vi "WS1033 Multi Socket HD Ver1.0.vi"() -> ()   [LabVIEW 2012]
uses:
  <vilib>/Utility/file.llb/Read From Spreadsheet File (DBL).vi
  _Employee_Folders/Andy temp/All Driver/agilent/Agilent E363X Series/Agilent E363X Series.lvlib
  _Employee_Folders/Andy temp/All Driver/Keithley/keithley_2000/Keithley 2000/Keithley 2000.lvlib
panel:
  out "Simulate FPGA":bool
  out "Online":bool
  out "PS1 Out":refnum<visa-resource-name>="GPIB0::5::INSTR"
  out "Ke2000 Out":refnum<visa-resource-name>="GPIB0::9::INSTR"
  in  "Reg3&4":string[](array[string])=["0600", "0601", "0600", "0602", "0600", "0604", "0600", "0608", "0600", "0610", "0600", "0620", "0600", "0640", "0600", "0801", "0800", "0802", "0800", "0804", "0800", "0808", "0800", "0810", "0800", "06FF", "0600", "08FF", "0800"]
  in  "VPI":string[](array[string])=["0200", "02FF", "0200", "04FF", "0400", "06FF", "0600", "08FF", "0800"]
  in  "VPI Drivers":string[](array[string])=["VPI_All_Drivers OFF", "VPI_Reg1_ON", "VPI_Reg1_OFF", "VPI_Reg2_ON", "VPI_Reg2_OFF", "VPI_Reg3_ON", "VPI_Reg3_OFF", "VPI_Reg4_ON", "VPI_Reg4_OFF"]
  in  "Tab Control":enum32{"Instrument Control", "Data Output"}(tab)
  in  "CP to Hold Down":T1(ring)
  in  "VPI Test":bool=TRUE
  in  "error in (no error)":errorcluster
  out "error out":errorcluster
  in  "Lot#":string="WS1033"
  in  "Wafer#":string="T4"
  in  "File Name":string="Test Data"
  in  "TMN DC\\CAP Data Log File Path":path=path "C:/Andy Temp/16 Socket"
  in  "SN":string[](array[string])=["010", "022", "03", "04", "05", "06", "070", "08", "09", "10", "112", "12", "13", "14", "15", "160"]
  in  "Test Program":string="Multi-Sockets HD/Cycling Ver1.0"
  out "Current Date":string="5/1/2013"
  out "Current Time":string="1517"
  in  "Start Date":string
  in  "Start Time":string
  in  "Comment":string="HD at 85C"
  in  "HD/Cycles":bool=TRUE
  in  "OK Button":bool
  in  "Calibration":bool
  in  "Verify CP":bool
  in  "VSA Test":bool
  in  "Reg1_Bit Cntrl":string[](array[string])=["1", "2", "4", "8", "10", "20", "40", "80", "3", "6", "C", "D8", "33", "66", "CC", "7", "E", "1C", "38", "70", "E0", "F", "1E", "3C", "78", "F0", "1F", "3E", "7C", "F8", "3F", "7E", "FC", "7F", "FE", "FD", "FB", "F7", "EF", "DF", "BF", "7F", "FC", "F9", "F3", "E7", "CF", "9F", "3F", "F8", "F1", "E3", "C7", "8F", "1F", "F0", "E1", "C3", "87", "F", "E0", "C1", "83", "7", "C0", "81", "3", "AA", "55", "0"]
  in  "PS1 Source":refnum<visa-resource-name>="GPIB0::5::INSTR"
  in  "Ke2000":refnum<visa-resource-name>="GPIB0::9::INSTR"
  in  "CP Setting":enum16{"CP OFF", "CP ON", "CP 35V", "CP 40V"}(ring)
  out "Cap_Data":string[][](table)=[["0x02", "-0.00078", "0x02", "-0.00036"], ["0x02", "0.00029", "0x00", "-8.19200"], ["0x02", "0.00068", "0x02", "0.00013"], ["0x02", "0.00009", "0x02", "1.40700"], ["0x02", "-0.00055", "0x02", "0.00020"], ["0x02", "-0.00045", "0x02", "-0.00050"], ["0x02", "0.00012", "0x02", "-0.00015"], ["0x02", "-0.00019", "0x02", "0.00001"], ["0x02", "0.00073", "0x02", "0.00026"], ["0x02", "-0.00007", "0x02", "0.00061"], ["0x02", "0.00030", "0x02", "-0.00042"], ["0x02", "-1.44418", "0x02", "-1.41436"], ["0x02", "-0.00019", "0x02", "0.00061"], ["0x02", "-0.00016", "0x02", "0.00049"], ["0x02", "-0.00066", "0x02", "-0.00044"], ["0x02", "0.00213", "0x02", "0.00170"]]
  out "Reg3&4":string[][](table)=[["-0.00084", "0.18754", "-0.00086", "0.18760", "-0.00067", "0.38012", "-0.00140", "0.75405", "-0.00094", "0.74436", "-0.00057", "0.74920", "-0.00020", "0.71688", "-0.00073", "0.10053", "-0.00077", "0.18613", "-0.00101", "0.37569", "-0.00052", "0.73663", "-0.00098", "0.71573", "-0.00100", "3.71894", "-0.00115", "2.11771", "-0.00113"], ["-8.19200", "-8.19200", "-8.19200", "-8.19200", "-8.19200", "-8.19200", "-8.19200", "-8.19200", "-8.19200", "-8.19200", "-8.19200", "-8.19200", "-8.19200", "-8.19200", "-8.19200", "-8.19200", "-8.19200", "-8.19200", "-8.19200", "-8.19200", "-8.19200", "-8.19200", "-8.19200", "-8.19200", "-8.19200", "-8.19200", "-8.19200", "-8.19200", "-8.19200"], ["0.00018", "0.24983", "0.00031", "0.25320", "0.00005", "0.40161", "0.00013", "0.84415", "-0.00005", "0.79338", "-0.00002", "0.89156", "-0.00008", "0.78759", "-0.00012", "0.12441", "0.00009", "0.23126", "0.00023", "0.44253", "-0.00006", "0.80303", "0.00005", "0.86221", "0.00024", "4.21607", "0.00055", "2.45958", "0.00055"], ["1.48104", "1.63231", "1.48088", "1.71195", "1.48077", "1.81328", "1.48126", "2.09433", "1.48064", "2.18596", "1.48090", "2.25438", "1.48055", "2.27741", "1.48033", "1.55337", "1.48025", "1.72992", "1.48041", "1.90426", "1.48006", "2.39045", "1.48012", "2.29779", "1.48036", "5.08456", "1.48139", "3.95496", "1.48067"], ["-0.00076", "0.23402", "-0.00052", "0.23805", "0.00035", "0.43666", "-0.00035", "0.84128", "-0.00062", "0.92223", "-0.00022", "0.94897", "-0.00033", "0.81247", "-0.00029", "0.09200", "-0.00033", "0.23124", "-0.00021", "0.40000", "-0.00052", "0.89413", "-0.00028", "0.85978", "0.00024", "4.43176", "0.00034", "2.47569", "0.00022"], ["0.00009", "0.18310", "-0.00025", "0.20594", "-0.00012", "0.36049", "-0.00083", "0.75674", "-0.00085", "0.80900", "0.00001", "0.77914", "-0.00048", "0.72434", "-0.00073", "0.10624", "-0.00040", "0.21135", "-0.00031", "0.39919", "-0.00078", "0.80036", "0.00025", "0.78208", "-0.00029", "3.81718", "-0.00030", "2.30191", "-0.00016"], ["0.00018", "0.23801", "0.00002", "0.20572", "0.00043", "0.45364", "0.00013", "0.85310", "0.00030", "0.88533", "0.00002", "0.86306", "0.00027", "0.90155", "0.00011", "0.11996", "0.00020", "0.20562", "0.00029", "0.38279", "-0.00007", "0.82877", "0.00010", "0.84844", "0.00000", "4.39414", "0.00041", "2.38263", "0.00046"], ["-0.00025", "-0.00033", "-0.00033", "-0.00005", "-0.00034", "-0.00020", "-0.00026", "-0.00016", "-0.00029", "-0.00028", "-0.00036", "-0.00026", "-0.00022", "0.00003", "-0.00031", "-0.00006", "-0.00004", "-0.00028", "-0.00012", "0.00002", "-0.00038", "-0.00007", "-0.00022", "-0.00013", "-0.00006", "0.00002", "0.00004", "-0.00006", "-0.00028"], ["-0.00024", "0.22994", "-0.00010", "0.20515", "0.00022", "0.35799", "0.00006", "0.85993", "0.00025", "0.49771", "-0.00013", "0.87203", "0.00013", "0.85128", "-0.00010", "0.10478", "-0.00009", "0.17132", "-0.00025", "0.27951", "0.00002", "0.88446", "-0.00001", "0.80268", "0.00025", "3.87229", "0.00045", "2.24245", "0.00032"], ["-0.00000", "0.21432", "0.00055", "0.22416", "0.00066", "0.46476", "0.00079", "0.82063", "0.00088", "0.91417", "0.00085", "0.71087", "0.00137", "0.88451", "0.00047", "0.12494", "0.00100", "0.21354", "0.00111", "0.39845", "0.00135", "0.87188", "0.00073", "0.83177", "0.00040", "4.22709", "0.00114", "2.43520", "0.00173"], ["0.00004", "0.21202", "0.00087", "0.18791", "-0.00050", "0.37207", "0.00000", "0.77774", "0.00003", "0.76047", "-0.00026", "0.73879", "0.00033", "0.74256", "0.00113", "0.09446", "-0.00033", "0.20280", "0.00057", "0.40386", "-0.00006", "0.74892", "0.00009", "0.75346", "0.00005", "3.78760", "-0.00022", "2.20027", "0.00007"], ["-1.38608", "-1.41365", "-1.38569", "-1.40262", "-1.41280", "-1.38552", "-1.38403", "-1.40605", "-1.41116", "-1.40218", "-1.38437", "-1.39281", "-1.41380", "-1.38576", "-1.41076", "-1.41382", "-1.38948", "-1.38451", "-1.40341", "-1.41316", "-1.38565", "-1.38617", "-1.41285", "-1.38543", "-1.39807", "-1.41301", "-1.38564", "-1.38315", "-1.41346"], ["-0.00011", "-0.00018", "-0.00016", "-0.00032", "0.00006", "0.00022", "-0.00012", "0.00029", "-0.00018", "-0.00014", "-0.00028", "-0.00016", "-0.00028", "-0.00043", "-0.00018", "-0.00058", "-0.00030", "-0.00043", "-0.00003", "-0.00086", "0.00001", "-0.00024", "-0.00032", "-0.00022", "-0.00052", "-0.00009", "-0.00015", "-0.00018", "-0.00010"], ["-0.28766", "-0.06844", "-0.28721", "-0.07378", "-0.28779", "0.09271", "-0.28773", "0.52467", "-0.28712", "0.47110", "-0.28710", "0.42933", "-0.31981", "0.48753", "-0.30479", "-0.19809", "-0.30441", "-0.09968", "-0.30354", "0.09009", "-0.30382", "0.49702", "-0.30349", "0.09602", "-0.30717", "3.60367", "-0.25810", "1.64223", "-0.25957"], ["-0.00059", "0.19570", "-0.00082", "0.20174", "0.00001", "0.39111", "-0.00072", "0.75114", "-0.00106", "0.76788", "-0.00014", "0.77680", "-0.00006", "0.76978", "-0.00018", "0.10645", "-0.00070", "0.20429", "-0.00002", "0.37780", "-0.00030", "0.81574", "-0.00013", "0.47817", "-0.00074", "3.85303", "-0.00048", "1.98246", "-0.00087"], ["0.00088", "0.20894", "-0.00005", "0.22869", "-0.00426", "0.43002", "0.00310", "0.90978", "-0.00419", "0.79785", "-0.00166", "0.91643", "0.00103", "0.78807", "0.00092", "0.11746", "-0.00434", "0.23011", "0.00081", "0.44810", "0.00235", "0.85701", "-0.00171", "0.69913", "-0.00388", "4.28342", "-0.00044", "2.35229", "0.00221"]]
  out "Reg1&2":string[][](table)=[["-0.00108", "0.08958", "-0.00053", "0.18959", "-0.00078", "0.37850", "-0.00171", "0.76297", "-0.00120", "0.76690", "-0.00101", "0.77762", "-0.00044", "0.77961", "-0.00083", "0.18983", "-0.00150", "0.19728", "-0.00157", "0.36782", "-0.00119", "0.75459", "-0.00103", "0.71258", "-0.00099", "3.74809", "-0.00130", "2.22378", "-0.00086"], ["-0.00041", "0.10906", "-0.00055", "0.19752", "-0.00042", "0.45314", "-0.00099", "0.87667", "-0.00092", "0.86594", "-0.00012", "0.87358", "-0.00063", "0.85050", "-0.00091", "0.19742", "-0.00169", "0.22081", "-0.00095", "0.43763", "-0.00006", "0.81361", "0.00021", "0.79624", "0.00004", "4.22385", "-0.00056", "2.46734", "0.00029"], ["-0.00071", "0.12205", "-0.00101", "0.23127", "-0.00120", "0.45826", "-0.00166", "0.76407", "-0.00138", "0.93942", "-0.00113", "0.85225", "-0.00202", "0.71053", "-0.00199", "0.18763", "-0.00186", "0.20697", "-0.00161", "0.45450", "-0.00214", "0.91461", "-0.00233", "0.89898", "-0.00220", "4.07969", "-0.00177", "2.66987", "-0.00206"], ["0.00302", "0.12120", "0.00300", "0.23274", "0.00271", "0.43565", "0.00310", "0.81019", "0.00284", "0.80161", "0.00285", "0.85918", "0.00327", "0.75798", "0.00290", "0.17085", "0.00258", "0.26002", "0.00243", "0.36001", "0.00210", "0.84827", "0.00265", "0.83634", "0.00302", "3.99829", "0.00392", "2.46160", "0.00326"], ["-0.00053", "0.10355", "0.00018", "0.23057", "-0.00018", "0.41330", "-0.00084", "0.85901", "-0.00029", "0.90795", "-0.00049", "0.86511", "-0.00023", "0.66685", "-0.00013", "0.20790", "-0.00045", "0.23230", "-0.00036", "0.36861", "-0.00021", "0.91175", "-0.00039", "0.89470", "-0.00022", "4.04444", "0.00030", "2.61219", "0.00067"], ["-0.00065", "0.10915", "-0.00041", "0.15397", "-0.00086", "0.40657", "-0.00049", "0.80189", "-0.00024", "0.79573", "-0.00090", "0.74982", "0.00009", "0.74729", "-0.00032", "0.20103", "-0.00066", "0.15526", "-0.00050", "0.35926", "-0.00085", "0.76617", "-0.00037", "0.73687", "-0.00084", "3.76376", "0.00006", "2.21866", "-0.00009"], ["0.00030", "0.12056", "0.00004", "0.20153", "0.00009", "0.42879", "0.00031", "0.89839", "0.00030", "0.70209", "0.00002", "0.88332", "-0.00002", "0.93653", "-0.00001", "0.23214", "0.00040", "0.24748", "0.00040", "0.38589", "-0.00015", "0.75535", "0.00037", "0.89693", "0.00052", "4.16809", "0.00050", "2.51317", "0.00018"], ["0.00012", "-0.00046", "-0.00024", "-0.00022", "-0.00021", "0.00039", "0.00039", "0.00026", "0.00009", "0.00010", "-0.00005", "0.00003", "-0.00016", "0.00013", "-0.00015", "0.00033", "0.00036", "0.00017", "0.00032", "0.00028", "0.00018", "0.00043", "-0.00002", "0.00009", "0.00019", "0.00002", "0.00005", "0.00006", "-0.00005"], ["0.00070", "0.11336", "0.00036", "0.21945", "-0.00001", "0.38795", "0.00026", "0.82826", "0.00041", "0.80312", "-0.00028", "0.40543", "0.00037", "0.75070", "0.00052", "0.18489", "-0.00025", "0.21492", "0.00034", "0.43130", "0.00022", "0.86169", "0.00032", "0.82752", "0.00056", "3.50231", "0.00059", "2.51767", "0.00054"], ["-0.00061", "0.09307", "-0.00031", "0.17837", "-0.00027", "0.43916", "-0.00046", "0.88525", "-0.00032", "0.82577", "-0.00056", "0.86653", "-0.00034", "0.90515", "-0.00020", "0.20958", "-0.00047", "0.20748", "-0.00045", "0.46265", "-0.00032", "0.90088", "-0.00056", "0.79231", "-0.00016", "4.19054", "0.00021", "2.57487", "0.00006"], ["0.00103", "0.10551", "0.00060", "0.20551", "0.00094", "0.32942", "0.00117", "0.71118", "0.00014", "0.76176", "0.00086", "0.80010", "0.00036", "0.75930", "0.00082", "0.18517", "0.00065", "0.21107", "0.00123", "0.37059", "0.00126", "0.74420", "-0.00022", "0.71578", "0.00077", "3.66523", "0.00031", "2.22177", "0.00081"], ["-1.42429", "-1.44113", "-1.41095", "-1.44427", "-1.44315", "-1.41113", "-1.41886", "-1.44365", "-1.44414", "-1.42234", "-1.41414", "-1.43293", "-1.44072", "-1.41408", "-1.44534", "-1.44074", "-1.41168", "-1.41344", "-1.44284", "-1.44325", "-1.41192", "-1.42341", "-1.44250", "-1.41447", "-1.43829", "-1.44336", "-1.41174", "-1.41548", "-1.44290"], ["-0.00040", "-0.00058", "-0.00069", "-0.00034", "-0.00091", "-0.00007", "-0.00026", "0.00017", "-0.00029", "-0.00053", "-0.00067", "-0.00019", "-0.00032", "-0.00082", "-0.00022", "-0.00101", "-0.00044", "-0.00060", "-0.00033", "-0.00070", "-0.00014", "-0.00033", "-0.00039", "-0.00033", "-0.00050", "-0.00045", "-0.00058", "-0.00057", "-0.00050"], ["0.26147", "0.37198", "0.26509", "0.37993", "0.26735", "0.61084", "0.27247", "1.16162", "0.35145", "0.37885", "0.19776", "0.31024", "0.20096", "0.87044", "0.12135", "0.33067", "0.12190", "0.31888", "0.12124", "0.49791", "0.12085", "0.83089", "0.11981", "0.90413", "0.12004", "2.33768", "0.36618", "2.64833", "0.37380"], ["-0.00125", "0.08024", "-0.00154", "0.18501", "-0.00112", "0.35777", "-0.00077", "0.79151", "-0.00136", "0.70398", "-0.00169", "0.76332", "-0.00093", "0.74859", "-0.00069", "0.17705", "-0.00076", "0.16984", "-0.00130", "0.38821", "-0.00132", "0.79636", "-0.00084", "0.74254", "-0.00106", "3.63462", "-0.00039", "2.27469", "-0.00088"], ["-0.00006", "0.10215", "0.00384", "0.20083", "-0.00340", "0.41008", "0.00403", "0.77711", "-0.00457", "0.89558", "0.00300", "0.84232", "0.00019", "0.89071", "0.00511", "0.24260", "-0.00298", "0.23605", "0.00029", "0.35134", "0.00335", "0.77986", "0.00245", "0.86336", "-0.00354", "4.12034", "-0.00111", "2.46775", "0.00576"]]
  out "STATUS":string="Idle...."
  in  "Set HD/Cycle \nto Complete":i16=2
  out "No of HD/Cycle\nCompleted":i16=2
  out "EFuse Readback Status":bool[](array[boolean])
  in  "stop During HD/Cycles":bool
  in  "stop":bool
  in  "Reg1&2":string[](array[string])=["0200", "0201", "0200", "0202", "0200", "0204", "0200", "0208", "0200", "0210", "0200", "0220", "0200", "0240", "0200", "0401", "0400", "0402", "0400", "0404", "0400", "0408", "0400", "0410", "0400", "02FF", "0200", "04FF", "0400"]
  in  "Drivers":string[](array[string])=["C1_1 & C2_1Min", "C1_D0 & C2_D12", "C1_D0 & C2_D12 OFF", "C1_D1 & C2_D13", "C1_D1 & C2_D13 OFF", "C1_D2 & C2_D14", "C1_D2 & C2_D14 OFF", "C1_D3 & C2_D15", "C1_D3 & C2_D15 OFF", "C1_D4 & C2_D16", "C1_D4 & C2_D16 OFF", "C1_D5 & C2_D17", "C1_D5 & C2_D17 OFF", "C1_D6 & C2_D18", "C1_D6 & C2_D18 OFF", "C1_D7 & C2_D19", "C1_D7 & C2_D19 OFF", "C1_D8 & C2_D20", "C1_D8 & C2_D20 OFF", "C1_D9 & C2_D21", "C1_D9 & C2_D21 OFF", "C1_D10 & C2_D22", "C1_D10 & C2_D22 OFF", "C1_D11 & C2_D23", "C1_D11 & C2_D23 OFF", "Reg1 & Reg3 ON", "Reg1 & Reg3 OFF", "Reg2 & Reg4 ON", "Reg2 & Reg4 OFF"]
  # "*********** Do Not Remove*******\nCompany:  WiSpry Inc\n20 Fairbanks Ste 198 Irvine CA 92618\n\nAuthor:  Andy V Tran\nCreated:  03/06/2013\nLabVIEW2009 Pro\nTest Program:  \nWS1033 Multi-Socket HD/Cycle ver1.0\n*******************************"
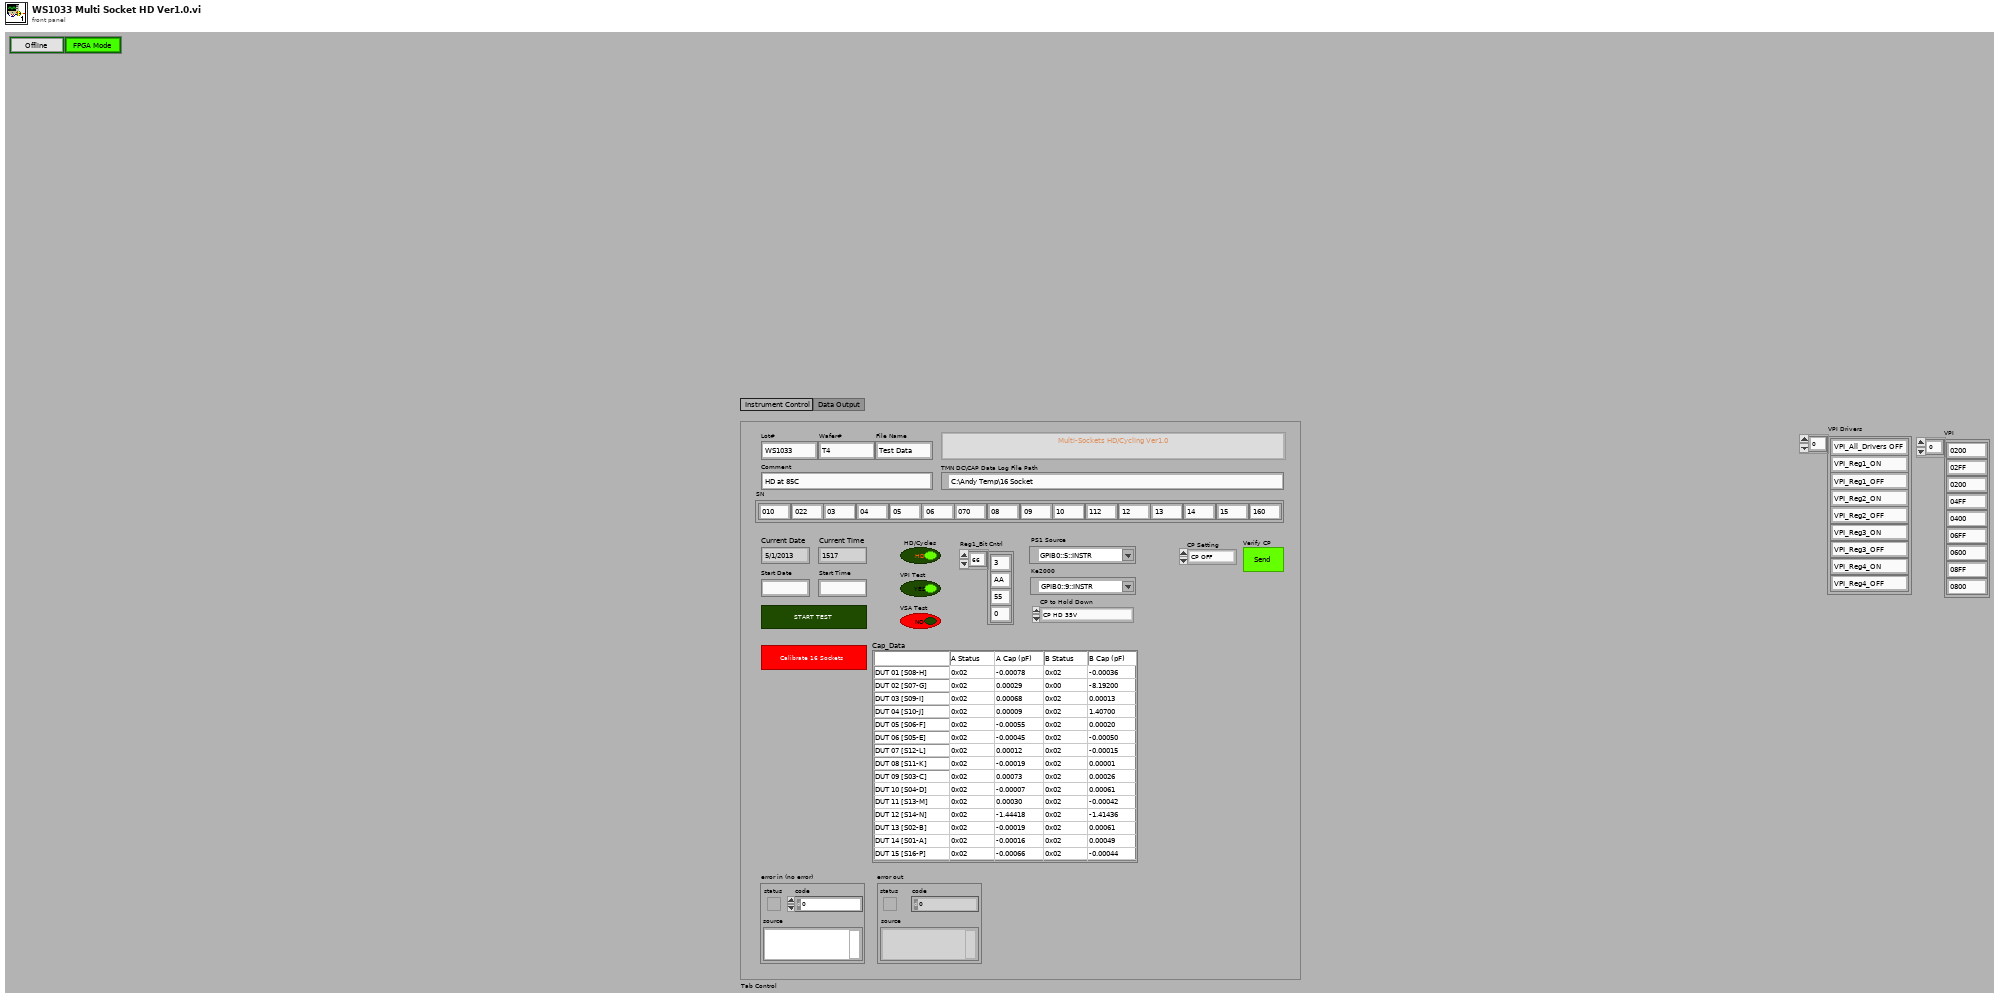
[diagram p1: front panel]
types:
  T1 = enum16{"CP HD 35V", "CP HD 40V", "CP HD 26V", "CP HD 30V"}
  T2 = typedef "WSVCAP SHL Core System Cluster.ctl" = cluster{"Settings":T3, "FPGA Resource":tag, "Online":bool}
  T3 = typedef "WSVCAP SHL I2C Settings Cluster.ctl" = cluster{"FPGA Resource Name":string, "I2C Slave Address":u8, "I2C Clock Rate (Hz)":dbl, "SPI Clock Rate (Hz)":dbl, "Simulate FPGA":bool}
  T4 = enum16{"Idle...", "Voltage 1", "Voltage 2", "Voltage 3"}[]
  T5 = cluster{"Test Program ":string, "Comment":string}
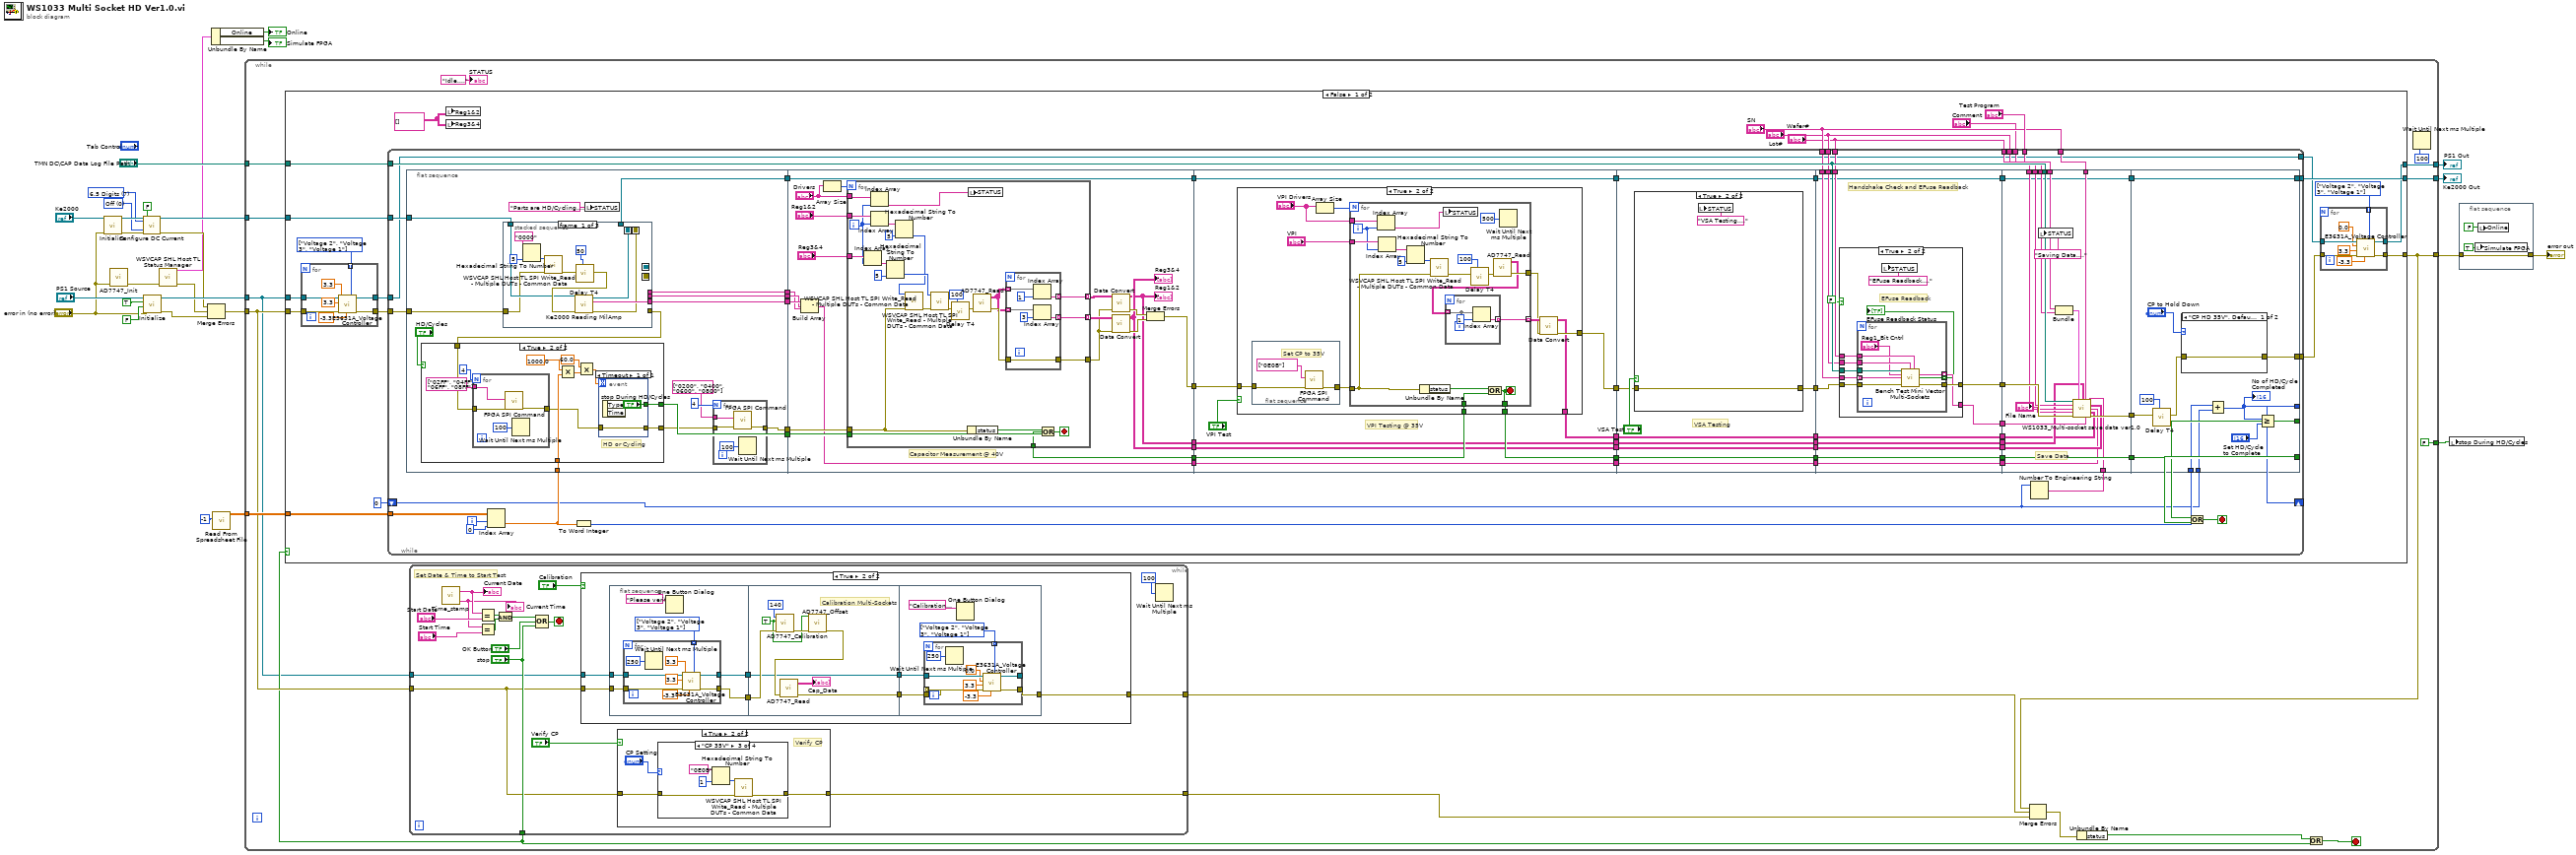
[diagram p0: block diagram]
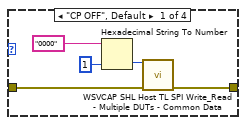
[diagram p3: hidden frame]
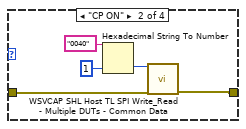
[diagram p4: hidden frame]
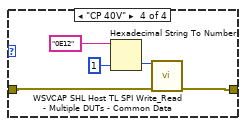
[diagram p5: hidden frame]
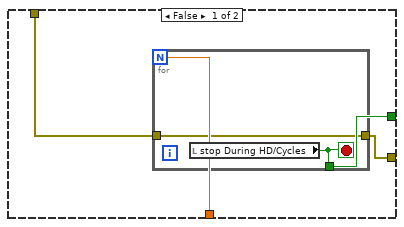
[diagram p7: hidden frame]
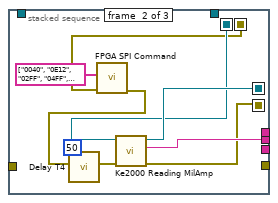
[diagram p8: hidden frame]
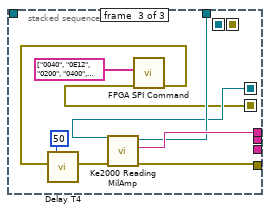
[diagram p9: hidden frame]
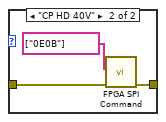
[diagram p13: hidden frame]
diagram:
  w17 = u16 0 items=["Off", "Moving Filter", "Repeating Filter"] ("Digital Filter (0: Off)")
  w18 = u16 7 items=["3.5 Digits"=4, "4.5 Digits"=5, "5.5 Digits"=6, "6.5 Digits"=7] ("Resolution (7: 6.5 digits)")
  n1 = call "Initialize.vi"("VISA resource name"="Ke2000", "error in (no error)"="error in (no error)") -> ("VISA resource name out"=w20:refnum<visa-resource-name>, "error out"=w19:errorcluster)  [unwired: 16 in]
  n2 = call "AD7747_Init.vi"("error in"="error in (no error)") -> ("error out"=w4:errorcluster)  [unwired: 10 in]
  n3 = call "Configure DC Current.vi"("VISA resource name"=w20, "Resolution (7: 6.5 digits)"=w18, "error in (no error)"=w19, "Auto Range? (T: Auto)"=FALSE, "Digital Filter (0: Off)"=w17) -> ("VISA resource name out"=w11:refnum<visa-resource-name>, "error out"=w14:errorcluster)  [unwired: 13 in]
  n4 = call "Initialize.vi"("error in (no error)"="error in (no error)", "Reset? (T: Yes)"=FALSE, "ID Query? (T: Yes)"=TRUE, "VISA resource name"="PS1 Source") -> ("error out"=w13:errorcluster, "VISA resource name out"=w23:refnum<visa-resource-name>)  [unwired: 6 in]
  n5 = call "WSVCAP SHL Host TL Status Manager.vi"("error in"=w4) -> ("System Out"=w7:T2, "error out"=w3:errorcluster)  [unwired: 13 in]
  n6 = Merge Errors(w14, w3, w13) -> (w12:errorcluster)
  n7 = Unbundle By Name(w7) -> ("Online"=→"Online":bool, "Settings.Simulate FPGA"=→"Simulate FPGA":bool)
  n8 = call-poly <vilib>:"Read From Spreadsheet File.vi"("number of rows (all:-1)"=-1) -> ("all rows"=w27:dbl[][])  [unwired: 6 in, 4 out]
  n9 = while {
    tunnel: w12 -> [w39]
    tunnel: [w37] -> w1
    tunnel: w27 -> [w42]
    tunnel: "TMN DC\\CAP Data Log File Path" -> [w41]
    tunnel: w23 -> [w33]
    tunnel: w11 -> [w32]
    tunnel: [w31] -> w10
    tunnel: [w30] -> w9
    tunnel: [FALSE ("stop During HD/Cycles")] -> w8
    stop <- w43 stop-if-true
    n10 = while {
      tunnel: ["stop"] -> w38
      tunnel: w39 -> [w49]
      tunnel: [w48] -> w36
      tunnel: [w47] -> w35
      tunnel: w33 -> [w46]
      stop <- w55 stop-if-true
      # "Set Date & Time to Start Test"
      n11 = call "Time_stamp.vi"() -> ("date/time string"=w60:string, "date string"=w62:string)  [unwired: 2 in]
      "Current Date" <- w62
      "Current Time" <- w60
      n12 = Equal?(x=w62, y="Start Date") -> (x = y?=w58:bool)
      n13 = Equal?(x=w60, y="Start Time") -> (x = y?=w57:bool)
      n14 = And(x=w58, y=w57) -> (x .and. y?=w54:bool)
      n15 = Compound Arithmetic op=OR(w54, "OK Button", "stop") -> (w55:bool)
      n16 = case shown="True" "Calibration" {
        tunnel: w49 -> [w87 w94]
        tunnel: [w87 w91] -> w48
        tunnel: w46 -> [_ w90]
        frame False {
        }
        frame True {
          n17 = flat-sequence {
            tunnel: w94 -> [w98]
            tunnel: [w97] -> w93
            tunnel: w90 -> [w96]
            tunnel: [w95] -> w89
            tunnel: w93 -> [w115]
            tunnel: [w112] -> w92
            tunnel: w89 -> [w110]
            tunnel: [w110] -> w88
            tunnel: w92 -> [w120]
            tunnel: [w121] -> w91
            tunnel: w88 -> [w119]
            frame #0 {
              w99 = T4 [enum."Voltage 2", enum."Voltage 3", enum."Voltage 1"] items=["Idle...", "Voltage 1", "Voltage 2", "Voltage 3"]
              n18 = for {
                tunnel: w98 -> [w109]
                tunnel: w96 -> [w108]
                tunnel: w99 -> [w104] mode=indexing
                tunnel: [w103] -> w97
                tunnel: [w102] -> w95
                n19 = Wait Until Next ms Multiple(millisecond multiple=u32 250) -> ()  [unwired: 1 out]
                n20 = call "E3631A_Voltage Controller.vi"("Channel Controller"=w104, "Voltage 3"=-3.3, "error in (no error)"=w109, "Voltage 2"=3.3, "Voltage 1"=3.3, "VISA resource name"=w108) -> ("error out"=w103:errorcluster, "VISA resource name out"=w102:refnum<visa-resource-name>)  [unwired: 4 in]
              }
              n21 = One Button Dialog(message="Please verify all sockets should be empty...") -> ()  [unwired: 1 in, 1 out]
            }
            frame #1 {
              w114 = TRUE ("Read After CapDac?")
              # "Calibration Multi-Sockets"
              n22 = call "AD7747_Calibration.vi"("error in"=w115, "Read After CapDac?"=w114, "Cap_Dac Value"=u8 140) -> ("errorout"=w116:errorcluster)  [unwired: 7 in, 1 out]
              n23 = call "AD7747_Offset.vi"("error in"=w116, "Read?"=w114) -> ("error Out"=w113:errorcluster)  [unwired: 8 in, 1 out]
              n24 = call "AD7747_Read.vi"("error in"=w113) -> ("error Out"=w112:errorcluster, "AD7747 Values"=→"Cap_Data":string[][])  [unwired: 3 in]
            }
            frame #2 {
              w118 = T4 [enum."Voltage 2", enum."Voltage 3", enum."Voltage 1"] items=["Idle...", "Voltage 1", "Voltage 2", "Voltage 3"]
              n25 = for {
                tunnel: [w124] -> _ mode=indexing
                tunnel: w119 -> [w131]
                tunnel: w118 -> [w123] mode=indexing
                tunnel: [w127] -> w121
                tunnel: [w126] -> _
                tunnel: w120 -> [w124]
                n26 = Wait Until Next ms Multiple(millisecond multiple=u32 250) -> ()  [unwired: 1 out]
                n27 = call "E3631A_Voltage Controller.vi"("Channel Controller"=w123, "Voltage 3"=-3.3, "error in (no error)"=w124, "Voltage 2"=3.3, "Voltage 1"=0.0, "VISA resource name"=w131) -> ("error out"=w127:errorcluster, "VISA resource name out"=w126:refnum<visa-resource-name>)  [unwired: 4 in]
              }
              n28 = One Button Dialog(message="Calibration Completed....") -> ()  [unwired: 1 in, 1 out]
            }
          }
        }
      }
      n29 = case shown="True" "Verify CP" {
        tunnel: w49 -> [w63 w66]
        tunnel: [w63 w65] -> w47
        frame False {
        }
        frame True {
          # "Verify CP"
          n30 = case shown="\"CP 35V\"" "CP Setting" {
            tunnel: w66 -> [w69 w74 w78 w83]
            tunnel: [w68 w73 w79 w84] -> w65
            frame "CP OFF", Default {
              n31 = Hexadecimal String To Number(string="0000" ("SPI Command"), default (0uL)=u16 1 ("default (0 U32)")) -> (number=w71:u16)  [unwired: 1 in, 1 out]
              n32 = call "WSVCAP SHL Host TL SPI Write_Read - Multiple DUTs - Common Data.vi"("Data Out [U64]"=w71, "error in"=w69) -> ("error out"=w68:errorcluster)  [unwired: 12 in, 1 out]
            }
            frame "CP ON" {
              n33 = Hexadecimal String To Number(string="0040" ("SPI Command"), default (0uL)=u16 1 ("default (0 U32)")) -> (number=w76:u16)  [unwired: 1 in, 1 out]
              n34 = call "WSVCAP SHL Host TL SPI Write_Read - Multiple DUTs - Common Data.vi"("Data Out [U64]"=w76, "error in"=w74) -> ("error out"=w73:errorcluster)  [unwired: 12 in, 1 out]
            }
            frame "CP 35V" {
              n35 = Hexadecimal String To Number(string="0E0B" ("SPI Command"), default (0uL)=u16 1 ("default (0 U32)")) -> (number=w81:u16)  [unwired: 1 in, 1 out]
              n36 = call "WSVCAP SHL Host TL SPI Write_Read - Multiple DUTs - Common Data.vi"("Data Out [U64]"=w81, "error in"=w78) -> ("error out"=w79:errorcluster)  [unwired: 12 in, 1 out]
            }
            frame "CP 40V" {
              n37 = Hexadecimal String To Number(string="0E12" ("SPI Command"), default (0uL)=u16 1 ("default (0 U32)")) -> (number=w86:u16)  [unwired: 1 in, 1 out]
              n38 = call "WSVCAP SHL Host TL SPI Write_Read - Multiple DUTs - Common Data.vi"("Data Out [U64]"=w86, "error in"=w83) -> ("error out"=w84:errorcluster)  [unwired: 12 in, 1 out]
            }
          }
        }
      }
      n39 = Wait Until Next ms Multiple(millisecond multiple=u32 100) -> ()  [unwired: 1 out]
    }
    n40 = case shown="False" w38 {
      tunnel: w39 -> [w144 w481]
      tunnel: [w133 w481] -> w37
      tunnel: w42 -> [w151 _]
      tunnel: w41 -> [w150 _]
      tunnel: w33 -> [w143 w479]
      tunnel: w32 -> [w140 w480]
      tunnel: [w139 w480] -> w31
      tunnel: [w135 w479] -> w30
      frame False {
        w132 = string[][] []
        w137 = T4 [enum."Voltage 2", enum."Voltage 3", enum."Voltage 1"] items=["Idle...", "Voltage 1", "Voltage 2", "Voltage 3"]
        w142 = T4 [enum."Voltage 2", enum."Voltage 3", enum."Voltage 1"] items=["Idle...", "Voltage 1", "Voltage 2", "Voltage 3"]
        n41 = for {
          tunnel: w144 -> [w168]
          tunnel: w143 -> [w167]
          tunnel: w142 -> [w163] mode=indexing
          tunnel: [w162] -> w141
          tunnel: [w161] -> w138
          n42 = call "E3631A_Voltage Controller.vi"("Channel Controller"=w163, "Voltage 3"=-3.3, "error in (no error)"=w168, "Voltage 2"=3.3, "Voltage 1"=3.3, "VISA resource name"=w167) -> ("error out"=w162:errorcluster, "VISA resource name out"=w161:refnum<visa-resource-name>)  [unwired: 4 in]
        }
        n43 = while {
          tunnel: w141 -> [w207]
          tunnel: [w223] -> w134
          tunnel: w151 -> [w230]
          shift-right: [w173] -> _
          shift-left: i16 0 -> [w169]
          tunnel: w150 -> [w217]
          tunnel: "Lot#" -> [w216]
          tunnel: "Wafer#" -> [w215]
          tunnel: "SN" -> [w214]
          tunnel: "Test Program" -> [w213]
          tunnel: "SN" -> [w212]
          tunnel: "Comment" -> [w211]
          tunnel: "Lot#" -> [w210]
          tunnel: "Wafer#" -> [w209]
          tunnel: w140 -> [w204]
          tunnel: [w198] -> w139
          tunnel: w138 -> [w197]
          tunnel: [w197] -> w136
          i -> [w228]
          stop <- w229 stop-if-true
          n44 = flat-sequence {
            tunnel: w170 -> [w245]
            tunnel: [w244] -> w226
            tunnel: w207 -> [w243]
            tunnel: [w234] -> w224
            tunnel: w204 -> [w239]
            tunnel: [w238] -> w203
            tunnel: [w237] -> w196
            tunnel: [w236] -> w195
            tunnel: [w235] -> w194
            tunnel: w226 -> [w320]
            tunnel: [w318] -> w192
            tunnel: w224 -> [w319]
            tunnel: [w305] -> w191
            tunnel: w203 -> [w314]
            tunnel: [w314] -> w190
            tunnel: w196 -> [w313]
            tunnel: w195 -> [w312]
            tunnel: w194 -> [w311]
            tunnel: [w304] -> w189
            tunnel: [w303] -> w188
            tunnel: [w302] -> w181
            tunnel: [w360] -> w222
            tunnel: [w359] -> w202
            tunnel: [w358] -> w193
            tunnel: w190 -> [w359]
            tunnel: w191 -> [w357]
            tunnel: w192 -> [w361]
            tunnel: w189 -> [w355]
            tunnel: w188 -> [w356]
            tunnel: [w356] -> w187
            tunnel: [w355] -> w186
            tunnel: w181 -> [w354]
            tunnel: [w354] -> w180
            tunnel: [w353] -> w176
            tunnel: w222 -> [w407]
            tunnel: [w407] -> w221
            tunnel: [w405] -> w219
            tunnel: w202 -> [w404]
            tunnel: [w404] -> w201
            tunnel: w193 -> [w403]
            tunnel: w187 -> [w402]
            tunnel: w186 -> [w401]
            tunnel: [w402] -> w185
            tunnel: [w401] -> w184
            tunnel: w180 -> [w400]
            tunnel: [w400] -> w179
            tunnel: w176 -> [w399]
            tunnel: [w399] -> w175
            tunnel: w221 -> [w424]
            tunnel: [w424] -> w220
            tunnel: w219 -> [w422]
            tunnel: [w421] -> w218
            tunnel: w217 -> [w423]
            tunnel: w216 -> [w420]
            tunnel: w215 -> [w419]
            tunnel: w214 -> [w418]
            tunnel: [w417] -> w208
            tunnel: w201 -> [w416]
            tunnel: [w416] -> w200
            tunnel: w185 -> [w414]
            tunnel: w184 -> [w413]
            tunnel: [w414] -> w183
            tunnel: [w413] -> w182
            tunnel: w179 -> [w412]
            tunnel: [w412] -> w178
            tunnel: w175 -> [w411]
            tunnel: [w411] -> w174
            tunnel: w220 -> [w462]
            tunnel: w218 -> [w461]
            tunnel: w217 -> [w459]
            tunnel: w213 -> [w453]
            tunnel: w212 -> [w457]
            tunnel: w211 -> [w452]
            tunnel: w210 -> [w456]
            tunnel: w209 -> [w451]
            tunnel: w208 -> [w454]
            tunnel: [w462] -> w206
            tunnel: [w460] -> w205
            tunnel: w200 -> [w449]
            tunnel: [w449] -> w199
            tunnel: w183 -> [w448]
            tunnel: w182 -> [w447]
            tunnel: w178 -> [w446]
            tunnel: w174 -> [w445]
            tunnel: w172 -> [w444]
            tunnel: [w465] -> w223
            tunnel: [w474] -> w225
            tunnel: w206 -> [w474]
            tunnel: w205 -> [w471]
            tunnel: w199 -> [w473]
            tunnel: [w473] -> w198
            tunnel: w171 -> [w469]
            tunnel: w169 -> [w468]
            tunnel: [w467] -> w173
            tunnel: [w466] -> w177
            frame #0 {
              n45 = stacked-sequence {
                seq-local: [w279 _ _] -> [_ w288 _]
                seq-local: [w278 _ _] -> [_ w289 _]
                seq-local: [_ w291 _] -> [_ _ w297]
                seq-local: [_ w290 _] -> [_ _ w298]
                tunnel: w243 -> [w273 _ _]
                tunnel: [_ _ w300] -> w242
                tunnel: [w283 _ _] -> w237
                tunnel: [_ w292 _] -> w236
                tunnel: [_ _ w301] -> w235
                tunnel: w239 -> [w280 _ _]
                tunnel: [_ _ w299] -> w238
                frame #0 {
                  n46 = Hexadecimal String To Number(string="0000" ("SPI Command"), default (0uL)=u32 5 ("default (0 U32)")) -> (number=w275:u32)  [unwired: 1 in, 1 out]
                  n47 = call "WSVCAP SHL Host TL SPI Write_Read - Multiple DUTs - Common Data.vi"("Data Out [U64]"=w275, "error in"=w273) -> ("error out"=w277:errorcluster)  [unwired: 12 in, 1 out]
                  n48 = call "Delay T4.vi"("milliseconds to wait"=u32 50, "error in (no error)"=w277) -> ("error out"=w281:errorcluster)  [unwired: 9 in]
                  n49 = call "Ke2000 Reading MilAmp.vi"("error in (no error)"=w281, "VISA resource name"=w280) -> ("error out"=w279:errorcluster, "uA"=w283:string, "VISA resource name out"=w278:refnum<visa-resource-name>)  [unwired: 7 in]
                }
                frame #1 {
                  n50 = call "FPGA SPI Command.vi"("error in"=w288, "Array"=string[] ["0040", "0E12", "02FF", "04FF", "06FF", "08FF"]) -> ("error out"=w285:errorcluster)  [unwired: 9 in]
                  n51 = call "Delay T4.vi"("milliseconds to wait"=u32 50, "error in (no error)"=w285) -> ("error out"=w286:errorcluster)  [unwired: 9 in]
                  n52 = call "Ke2000 Reading MilAmp.vi"("error in (no error)"=w286, "VISA resource name"=w289) -> ("error out"=w291:errorcluster, "uA"=w292:string, "VISA resource name out"=w290:refnum<visa-resource-name>)  [unwired: 7 in]
                }
                frame #2 {
                  n53 = call "FPGA SPI Command.vi"("error in"=w297, "Array"=string[] ["0040", "0E12", "0200", "0400", "0600", "0800"]) -> ("error out"=w293:errorcluster)  [unwired: 9 in]
                  n54 = call "Delay T4.vi"("milliseconds to wait"=u32 50, "error in (no error)"=w293) -> ("error out"=w294:errorcluster)  [unwired: 9 in]
                  n55 = call "Ke2000 Reading MilAmp.vi"("error in (no error)"=w294, "VISA resource name"=w298) -> ("error out"=w300:errorcluster, "uA"=w301:string, "VISA resource name out"=w299:refnum<visa-resource-name>)  [unwired: 7 in]
                }
              }
              n56 = case shown="True" "HD/Cycles" {
                tunnel: w245 -> [w253 w266]
                tunnel: [w250 w261] -> w244
                tunnel: w242 -> [w252 w259]
                tunnel: [w251 w260] -> w233
                frame False {
                  n57 = for {
                    N: w253 -> [_]
                    tunnel: w252 -> [w255]
                    tunnel: [w255] -> w251
                    tunnel: [w254] -> w250
                    stop <- w254 stop-if-true
                    n58 = local read "stop During HD/Cycles"() -> (w254:bool)
                  }
                }
                frame True {
                  # "HD or Cycling"
                  n59 = for {
                    N: 4 -> [_]
                    tunnel: w259 -> [w268]
                    tunnel: [w269] -> w258
                    tunnel: string[] ["02FF", "04FF", "06FF", "08FF"] -> [w267]
                    n60 = call "FPGA SPI Command.vi"("error in"=w268, "Array"=w267) -> ("error out"=w269:errorcluster)  [unwired: 9 in]
                    n61 = Wait Until Next ms Multiple(millisecond multiple=u32 100) -> ()  [unwired: 1 out]
                  }
                  n62 = Multiply(x=1000.0, y=w266) -> (x*y=w264:dbl)
                  n63 = Multiply(x=60.0, y=w264) -> (x*y=w262:dbl)
                  n64 = event shown="[0] Timeout" {
                    selector: _ -> [_]
                    dyn-events: _ -> [_]
                    timeout: w262 -> [_]
                    tunnel: ["stop During HD/Cycles"] -> w261
                    tunnel: w258 -> [w271]
                    tunnel: [w271] -> w260
                    event Timeout {
                      n65 = event-data() -> ()  [unwired: 1 in, 2 out]
                    }
                  }
                }
              }
              n66 = local write "STATUS"("Parts are HD/Cycling...." ("STATUS")) -> ()
              n67 = for {
                N: 4 -> [_]
                tunnel: w233 -> [w247]
                tunnel: [w248] -> w234
                tunnel: string[] ["0200", "0400", "0600", "0800"] -> [w246]
                n68 = call "FPGA SPI Command.vi"("error in"=w247, "Array"=w246) -> ("error out"=w248:errorcluster)  [unwired: 9 in]
                n69 = Wait Until Next ms Multiple(millisecond multiple=u32 100) -> ()  [unwired: 1 out]
              }
            }
            frame #1 {
              # "Capacitor Measurement @ 40V"
              n70 = Build Array(w313, w312, w311) -> (w302:string[])
              n71 = Array Size(array="Drivers") -> (size(s)=w321:i32)
              n72 = for {
                N: w321 -> [_]
                tunnel: w319 -> [w335]
                tunnel: "Drivers" -> [w345]
                tunnel: "Reg1&2" -> [w343]
                tunnel: w320 -> [w341]
                tunnel: [w340] -> w318
                tunnel: "Reg3&4" -> [w333]
                tunnel: [w325] -> w308
                tunnel: [w323] -> w310 mode=indexing
                tunnel: [w322] -> w309 mode=indexing
                i -> [w332]
                stop <- w340 stop-if-true
                n73 = Index Array(array=w333, index=w332) -> (element=w334:string)
                n74 = Index Array(array=w345, index=w332) -> (element=w344:string)
                n75 = Index Array(array=w343, index=w332) -> (element=w339:string)
                n76 = Hexadecimal String To Number(string=w334, default (0uL)=u32 5 ("default (0 U32)")) -> (number=w336:u32)  [unwired: 1 in, 1 out]
                n77 = Hexadecimal String To Number(string=w339, default (0uL)=u16 5 ("default (0 U32)")) -> (number=w328:u16)  [unwired: 1 in, 1 out]
                n78 = call "WSVCAP SHL Host TL SPI Write_Read - Multiple DUTs - Common Data.vi"("Data Out [U64]"=w328, "error in"=w335) -> ("error out"=w331:errorcluster)  [unwired: 12 in, 1 out]
                n79 = call "WSVCAP SHL Host TL SPI Write_Read - Multiple DUTs - Common Data.vi"("Data Out [U64]"=w336, "error in"=w331) -> ("error out"=w329:errorcluster)  [unwired: 12 in, 1 out]
                n80 = call "Delay T4.vi"("milliseconds to wait"=u32 100, "error in (no error)"=w329) -> ("error out"=w338:errorcluster)  [unwired: 9 in]
                n81 = Unbundle By Name(w335) -> ("status"=w342:bool)
                n82 = local write "STATUS"(w344) -> ()
                n83 = call "AD7747_Read.vi"("error in"=w338) -> ("error Out"=w326:errorcluster, "AD7747 Values"=w324:string[][])  [unwired: 3 in]
                n84 = for {
                  tunnel: w324 -> [w351] mode=indexing
                  tunnel: w326 -> [w352]
                  tunnel: [w352] -> w325
                  tunnel: w324 -> [w349] mode=indexing
                  tunnel: [w348] -> w322 mode=indexing
                  tunnel: [w346] -> w323 mode=indexing
                  n85 = Index Array(array=w351, index=1) -> (element=w346:string)
                  n86 = Index Array(array=w349, index=3) -> (element=w348:string)
                }
                n87 = Or(x=w342, y=w341) -> (x .or. y?=w340:bool)
              }
              n88 = call "Data Convert.vi"("error in (no error)"=w308, "Array 2"=w310) -> ("error out"=w307:errorcluster, "Data Out"=w303:string[][])  [unwired: 8 in]
              "Reg1&2" <- w303
              n89 = call "Data Convert.vi"("error in (no error)"=w308, "Array 2"=w309) -> ("error out"=w306:errorcluster, "Data Out"=w304:string[][])  [unwired: 8 in]
              "Reg3&4" <- w304
              n90 = Merge Errors(w307, w306) -> (w305:errorcluster)
            }
            frame #2 {
              # "VPI Testing @ 35V"
              n91 = case shown="True" "VPI Test" {
                tunnel: w361 -> [_ w371]
                tunnel: [_ w370] -> w360
                tunnel: [w363 w365] -> w358
                tunnel: w357 -> [w363 w368]
                tunnel: [_ w364] -> w353
                frame False {
                }
                frame True {
                  n92 = flat-sequence {
                    tunnel: [w377] -> w369
                    tunnel: w368 -> [w376]
                    frame #0 {
                      # "Set CP to 35V"
                      n93 = call "FPGA SPI Command.vi"("error in"=w376, "Array"=string[] ["0E0B"]) -> ("error out"=w377:errorcluster)  [unwired: 9 in]
                    }
                  }
                  n94 = Array Size(array="VPI Drivers") -> (size(s)=w374:i32)
                  n95 = for {
                    N: w374 -> [_]
                    tunnel: "VPI Drivers" -> [w395]
                    tunnel: "VPI" -> [w393]
                    tunnel: w369 -> [w382]
                    tunnel: w371 -> [w390]
                    tunnel: [w389] -> w370
                    tunnel: [w381] -> w366
                    tunnel: [w378] -> w367 mode=indexing
                    i -> [w380]
                    stop <- w389 stop-if-true
                    n96 = Index Array(array=w395, index=w380) -> (element=w394:string)
                    n97 = Index Array(array=w393, index=w380) -> (element=w383:string)
                    n98 = Hexadecimal String To Number(string=w383, default (0uL)=u16 5 ("default (0 U32)")) -> (number=w385:u16)  [unwired: 1 in, 1 out]
                    n99 = Unbundle By Name(w382) -> ("status"=w391:bool)
                    n100 = call "WSVCAP SHL Host TL SPI Write_Read - Multiple DUTs - Common Data.vi"("Data Out [U64]"=w385, "error in"=w382) -> ("error out"=w386:errorcluster)  [unwired: 12 in, 1 out]
                    n101 = local write "STATUS"(w394) -> ()
                    n102 = call "Delay T4.vi"("milliseconds to wait"=u32 100, "error in (no error)"=w386) -> ("error out"=w387:errorcluster)  [unwired: 9 in]
                    n103 = Or(x=w391, y=w390) -> (x .or. y?=w389:bool)
                    n104 = call "AD7747_Read.vi"("error in"=w387) -> ("error Out"=w381:errorcluster, "AD7747 Values"=w379:string[][])  [unwired: 3 in]
                    n105 = for {
                      tunnel: [w396] -> _ mode=indexing
                      tunnel: [w397] -> w378 mode=indexing
                      tunnel: w379 -> [w396] mode=indexing
                      n106 = Index Array(array=w396, index=1) -> (element=w397:string)
                    }
                    n107 = Wait Until Next ms Multiple(millisecond multiple=u32 500) -> ()  [unwired: 1 out]
                  }
                  n108 = call "Data Convert.vi"("error in (no error)"=w366, "Array 2"=w367) -> ("error out"=w365:errorcluster, "Data Out"=w364:string[][])  [unwired: 8 in]
                }
              }
            }
            frame #3 {
              # "VSA Testing"
              n109 = case shown="True" "VSA Test" {
                tunnel: w403 -> [w408 w410]
                tunnel: [w408 w410] -> w405
                frame False {
                }
                frame True {
                  n110 = local write "STATUS"("VSA Testing...." ("STATUS")) -> ()
                }
              }
            }
            frame #4 {
              # "Handshake Check and EFuse Readback"
              # "EFuse Readback"
              n111 = case shown="True" FALSE {
                tunnel: w423 -> [_ w434]
                tunnel: w422 -> [w425 w433]
                tunnel: [w425 w432] -> w421
                tunnel: w420 -> [_ w431]
                tunnel: w419 -> [_ w430]
                tunnel: w418 -> [_ w429]
                tunnel: [_ w428] -> w417
                frame False {
                }
                frame True {
                  n112 = for {
                    tunnel: w434 -> [w443]
                    tunnel: w433 -> [w442]
                    tunnel: [w441] -> w432
                    tunnel: w431 -> [w440]
                    tunnel: w430 -> [w439]
                    tunnel: w429 -> [w438] mode=indexing
                    tunnel: [w437] -> w428 mode=indexing
                    tunnel: [w436] -> w427 mode=indexing
                    n113 = call "Bench Test Mini Vector Multi-Sockets.vi"("file path (use dialog)"=w443, "Lot #"=w440, "Wafer #"=w439, "Reg1_Bit Cntrl"="Reg1_Bit Cntrl", "SN #"=w438, "error"=w442) -> ("s? t:f"=w437:string, "P/F"=w436:bool, "error out"=w441:errorcluster)  [unwired: 6 in, 1 out]
                  }
                  "EFuse Readback Status" <- w427
                  n114 = local write "STATUS"("EFuse Readback...." ("STATUS")) -> ()
                }
              }
            }
            frame #5 {
              # "Save Data"
              n115 = local write "STATUS"("Saving Data...." ("STATUS")) -> ()
              n116 = Bundle("Test Program"=w453, "Comment"=w452) -> (w458:T5)  [unwired: 1 in]
              n117 = call "WS1033_Multi-socket save data ver1.0.vi"("TMN DC\\CAP Data Log File Path"=w459, "TP/Comment"=w458, "Data Output Reg1&2"=w448, "SN"=w457, "HD/Cycles Completed"=w444, "Lot#"=w456, "Data Output Reg3&4"=w447, "Wafer#"=w451, "Current"=w446, "File Name"="File Name", "VPI Out"=w445, "error in"=w461, "R/W Status"=w454) -> ("error out"=w460:errorcluster)  [unwired: 2 in]
            }
            frame #6 {
              n118 = call "Delay T4.vi"("milliseconds to wait"=u32 100, "error in (no error)"=w471) -> ("error out"=w464:errorcluster)  [unwired: 9 in]
              n119 = case shown="\"CP HD 35V\", Default" "CP to Hold Down" {
                tunnel: [w475 w478] -> w465
                tunnel: w464 -> [w475 w477]
                frame "CP HD 35V", Default {
                }
                frame "CP HD 40V" {
                  n120 = call "FPGA SPI Command.vi"("error in"=w477, "Array"=string[] ["0E0B"]) -> ("error out"=w478:errorcluster)  [unwired: 9 in]
                }
              }
              n121 = Add(x=w469, y=w468) -> (x+y=w467:i16)
              "No of HD/Cycle\nCompleted" <- w467
              n122 = Greater Or Equal?(x=w467, y="Set HD/Cycle \nto Complete") -> (x >= y?=w466:bool)
            }
          }
          n123 = Index Array(array=w230, index (row)=w228, index (col)=0 ("disabled index (col)")) -> (element=w170:dbl)
          n124 = To Word Integer(number=w170) -> (16bit integer=w171:i16)
          n125 = Number To Engineering String(4:w169) -> (0:w172:string)  [unwired: 3 in]
          n126 = Or(x=w177, y=w225) -> (x .or. y?=w229:bool)
        }
        n127 = local write "Reg1&2"(w132) -> ()
        n128 = local write "Reg3&4"(w132) -> ()
        n129 = for {
          tunnel: w134 -> [w160]
          tunnel: w136 -> [w159]
          tunnel: w137 -> [w155] mode=indexing
          tunnel: [w154] -> w133
          tunnel: [w153] -> w135
          n130 = call "E3631A_Voltage Controller.vi"("Channel Controller"=w155, "Voltage 3"=-3.3, "error in (no error)"=w160, "Voltage 2"=3.3, "Voltage 1"=0.0, "VISA resource name"=w159) -> ("error out"=w154:errorcluster, "VISA resource name out"=w153:refnum<visa-resource-name>)  [unwired: 4 in]
        }
      }
      frame True {
      }
    }
    n131 = Merge Errors(w37, w36, w35) -> (w34:errorcluster)
    n132 = Unbundle By Name(w34) -> ("status"=w44:bool)
    n133 = Or(x=w44, y=w38) -> (x .or. y?=w43:bool)
    n134 = Wait Until Next ms Multiple(millisecond multiple=u32 100) -> ()  [unwired: 1 out]
    "STATUS" <- "Idle...." ("STATUS")
  }
  "Ke2000 Out" <- w10
  "PS1 Out" <- w9
  n135 = local write "stop During HD/Cycles"(w8) -> ()
  n136 = flat-sequence {
    tunnel: w1 -> [w484]
    tunnel: [w484] -> w2
    frame #0 {
      n137 = local write "Simulate FPGA"(TRUE ("Online")) -> ()
      n138 = local write "Online"(FALSE ("Online")) -> ()
    }
  }
  "error out" <- w2
